vi "proyecto lrm.vi"() -> ()   [LabVIEW 2017]
uses:
  <vilib>/Analysis/baseanly.llb/Mean (DBL).vi
  <vilib>/Analysis/2dsp.llb/Real FFT.vi
  <vilib>/Instr/_visa.llb/VISA Configure Serial Port (Instr).vi
  <vilib>/Analysis/NI_AALPro.lvlib
  <vilib>/Analysis/NI_AALBase.lvlib
  <vilib>/LabVIEW Interface for Arduino/LabVIEW Interface for Arduino.lvlib
panel:
  out "frecuencia muscular":dbl
  out "XY Graph":cluster{"Y":dbl[], "Y":dbl[]}[](graph)
  in  "VISA resource":refnum<visa-resource-name>
  in  "stop":bool
  out "REGISTRO DE ELECTROMIOGRAFÍA":i32(graph)
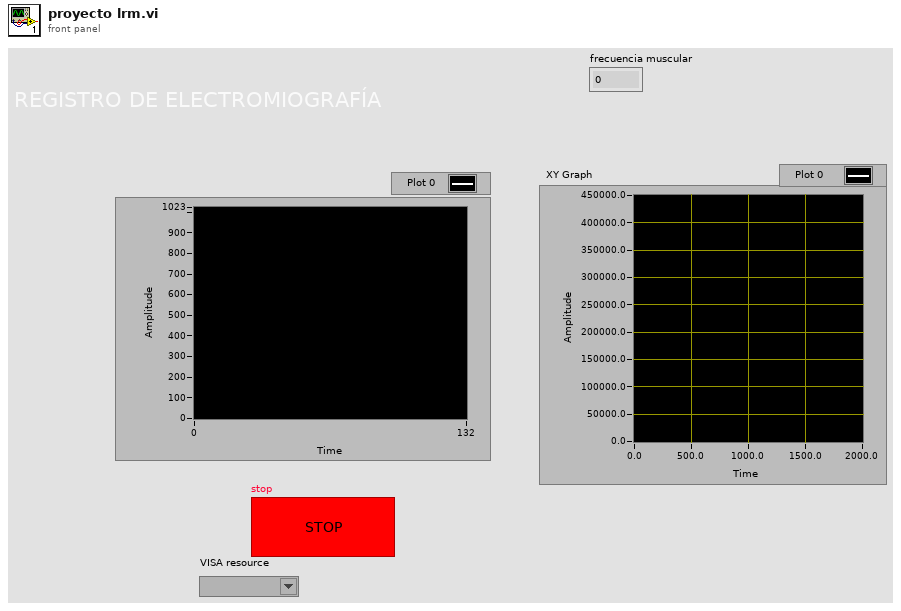
[diagram p1: front panel]
types:
  T1 = typedef "LabVIEW Interface for Arduino.lvlib/Arduino Resource.ctl" = cluster{"VISA resource":refnum<visa-resource-name>, "Board Type":T2, "Connection Type":enum8{"USB / Serial"}, "Bytes Per Packet (15)":u8}
  T2 = typedef "LabVIEW Interface for Arduino.lvlib/Board Type.ctl" = enum16{"Uno", "Dimuelanove w/Atmega 328", "Mega 2560"}
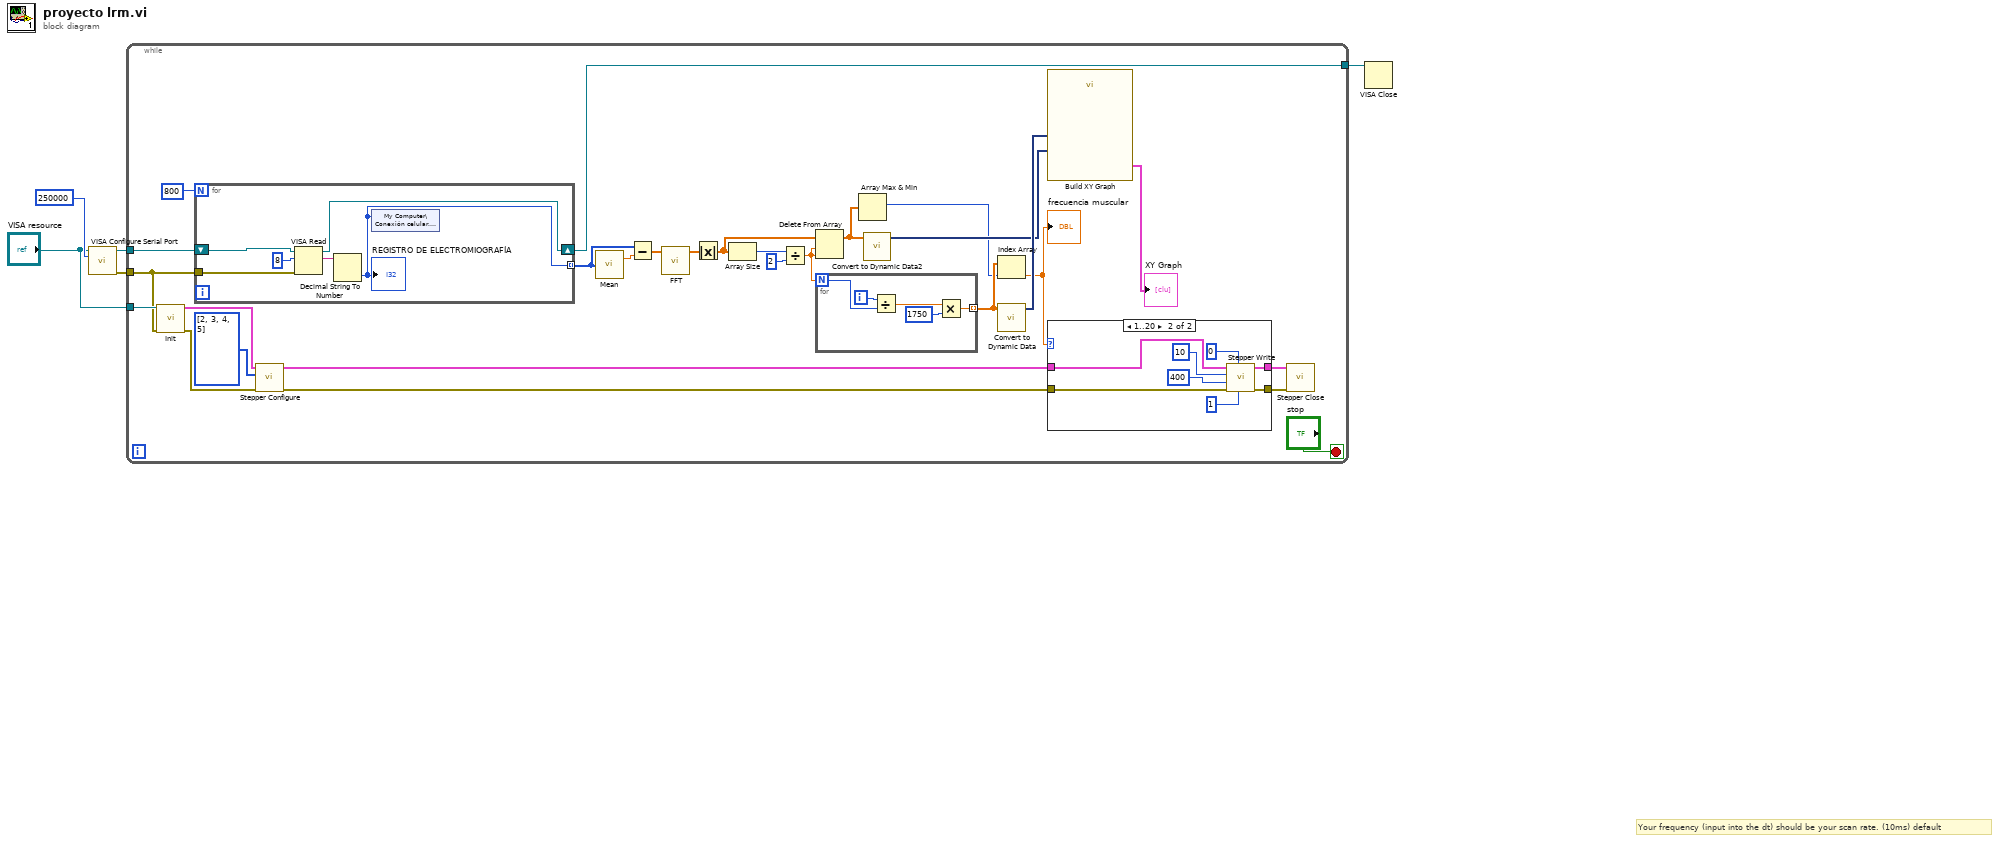
[diagram p0: block diagram]
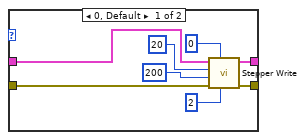
[diagram p2: hidden frame]
diagram:
  # "Your frequency (input into the dt) should be your scan rate. (10ms) default"
  n1 = call-poly "VISA Configure Serial Port"("VISA resource name"="VISA resource", "baud rate (9600)"=u32 250000) -> ("VISA resource name out"=w4:refnum<visa-resource-name>, "error out"=w3:errorcluster)  [unwired: 12 in]
  n2 = while {
    tunnel: w4 -> [w33]
    tunnel: w3 -> [w13]
    tunnel: [w16] -> w2
    tunnel: "VISA resource" -> [w14]
    stop <- "stop" stop-if-true
    n3 = call <vilib>:"Init.vi"("VISA resource"=w14, "error in"=w13) -> ("Arduino Resource"=w12:T1, "error out"=w11:errorcluster)  [unwired: 16 in]
    n4 = for {
      N: 800 -> [_]
      tunnel: w13 -> [w59]
      tunnel: [w55] -> w22 mode=indexing
      shift-right: [w56] -> w16
      shift-left: w33 -> [w60]
      n5 = VISA Read(VISA resource name=w60, byte count=u32 8, error in (no error)=w59) -> (VISA resource name out=w56:refnum<visa-resource-name>, read buffer=w57:string)  [unwired: 2 out]
      n6 = Decimal String To Number(string=w57) -> (number=w55:i32)  [unwired: 2 in, 1 out]
      "REGISTRO DE ELECTROMIOGRAFÍA" <- w55
      n7 = shared-variable "My Computer\\Conexión celular.lvlib\\emg3"(w55) -> ()  [unwired: 1 in, 1 out]
    }
    n8 = call <vilib>:"Stepper Configure.vi"("error in"=w11, "Stepper Pins"=u8[] [2, 3, 4, 5], "Arduino Resource"=w12) -> ("error out"=w8:errorcluster, "Arduino Resource Out"=w9:T1)  [unwired: 7 in]
    n9 = call-poly <vilib>:"Mean.vi"("X"=w22) -> ("mean"=w21:dbl)  [unwired: 1 out]
    n10 = Subtract(x=w22, y=w21) -> (x-y=w20:dbl[])
    n11 = call-poly <vilib>:"FFT.vi"("X"=w20) -> ("FFT {X}"=w30:cdb[])  [unwired: 9 in, 1 out]
    n12 = Absolute Value(x=w30) -> (abs(x)=w29:dbl[])
    n13 = Array Size(array=w29) -> (size(s)=w28:i32)
    n14 = Divide(x=w28, y=2) -> (x/y=w26:dbl)
    n15 = Delete From Array(array=w29, length=w26, index=w26) -> (array with subset deleted=w19:dbl[])  [unwired: 1 out]
    n16 = for {
      N: w26 -> [w51]
      tunnel: [w52] -> w18 mode=indexing
      i -> [w50]
      n17 = Divide(x=w50, y=w51) -> (x/y=w54:dbl)
      n18 = Multiply(x=w54, y=1750) -> (x*y=w52:dbl)
    }
    n19 = Array Max & Min(array=w19) -> (max index (indices)=w17:i32)  [unwired: 3 out]
    n20 = call "Convert to Dynamic Data2"("Array"=w19) -> ("Dynamic Data Type"=w23:dynamicdata)  [unwired: 3 in]
    n21 = Index Array(array=w18, index=w17) -> (element=w15:dbl)
    "frecuencia muscular" <- w15
    n22 = call "Convert to Dynamic Data"("Array"=w18) -> ("Dynamic Data Type"=w24:dynamicdata)  [unwired: 3 in]
    n23 = call "Build XY Graph"("Y Input"=w23, "X Input"=w24) -> ("XY Graph"=→"XY Graph":cluster{"X":dbl[], "Y":dbl[]}[])  [unwired: 8 in, 1 out]
    n24 = case shown="1..20" w15 {
      tunnel: w9 -> [w41 w46]
      tunnel: w8 -> [w40 w44]
      tunnel: [w35 w43] -> w7
      tunnel: [w34 w42] -> w6
      frame 0, Default {
        n25 = call <vilib>:"Stepper Write.vi"("Set Acceleration (0 to disable)"=i16 2, "Stepper #"=u8 0, "error in"=w40, "Set Speed (Steps per Second)"=i16 200, "# of Steps to Move"=i16 20, "Arduino Resource"=w41) -> ("error out"=w34:errorcluster, "Arduino Resource Out"=w35:T1)  [unwired: 4 in]
      }
      frame 1..20 {
        n26 = call <vilib>:"Stepper Write.vi"("Set Acceleration (0 to disable)"=i16 1, "Stepper #"=u8 0, "error in"=w44, "Set Speed (Steps per Second)"=i16 400, "# of Steps to Move"=i16 10, "Arduino Resource"=w46) -> ("error out"=w42:errorcluster, "Arduino Resource Out"=w43:T1)  [unwired: 4 in]
      }
    }
    n27 = call <vilib>:"Stepper Close.vi"("error in"=w6, "Arduino Resource"=w7) -> ()  [unwired: 8 in, 2 out]
  }
  n28 = VISA Close(VISA resource name=w2) -> ()  [unwired: 1 in, 1 out]
